vi "Do Request.vi"(7 "Processing In":refnum<class "Processing.lvclass">, 11 "CSRF in":refnum<class "CSRF.lvclass">) -> (0 "error out":errorcluster, 5 "Processing":refnum<class "Processing.lvclass">)   [LabVIEW 2020, in "Summer of LabVIEW.lvlib" / "CSRF.lvclass"]
uses:
  CSRF.lvclass
  <vilib>/IlluminatedG/IG HTTP Server/HTTP Server/Processing/Processing.lvclass
  CSRF.lvclass/CSRF.ctl
  <vilib>/IlluminatedG/IG HTTP Utils/HTTP Utils/Request/Request.lvclass
  <vilib>/IlluminatedG/IG HTTP Server/HTTP Server/HTTP Server.lvlib
  <vilib>/IlluminatedG/IG HTTP Utils/HTTP Utils/Response/Response.lvclass
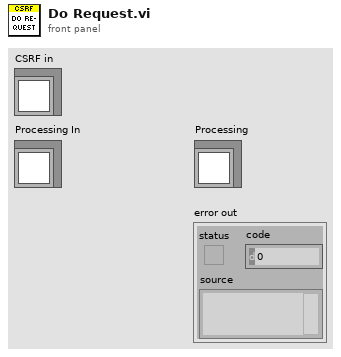
[diagram p1: front panel]
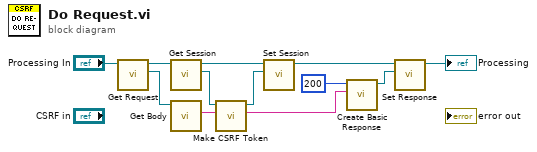
[diagram p0: block diagram]
diagram:
  n1 = call <vilib>:"Get Request.vi"("Processing in"="Processing In") -> ("Request"=w11:refnum<class "Request.lvclass">, "Processing out"=w10:refnum<class "Processing.lvclass">)  [unwired: 9 in]
  n2 = call <vilib>:"Get Session.vi"("Processing in"=w10) -> ("Session"=w9:refnum<class "Session.lvclass">, "Processing out"=w4:refnum<class "Processing.lvclass">)  [unwired: 9 in]
  n3 = call <vilib>:"Get Body.vi"("Request in"=w11) -> ("Body"=w8:string)  [unwired: 8 in, 2 out]
  n4 = call <vilib>:"Make CSRF Token.vi"("Token ID"=w8, "Session In"=w9) -> ("Token"=w2:string, "Session"=w3:refnum<class "Session.lvclass">)  [unwired: 7 in, 1 out]
  n5 = call <vilib>:"Set Session.vi"("Session"=w3, "Processing in"=w4) -> ("Processing out"=w1:refnum<class "Processing.lvclass">)  [unwired: 9 in]
  n6 = call <vilib>:"Create Basic Response.vi"("Payload"=w2, "Status Code"=u16 200) -> ("Response out"=w6:refnum<class "Response.lvclass">)  [unwired: 8 in, 1 out]
  n7 = call <vilib>:"Set Response.vi"("Response"=w6, "Processing in"=w1) -> ("Processing out"=→"Processing":refnum<class "Processing.lvclass">)  [unwired: 9 in]
